vi "I64 to ZigZag.vi"(11 "sint64":i64) -> (3 "ZigZag I64":i64)   [LabVIEW 2020, in "LV-Proto.lvlib"]
uses:
  LV-Proto.lvlib
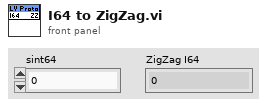
[diagram p1: front panel]
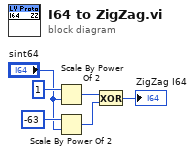
[diagram p0: block diagram]
diagram:
  n1 = Scale By Power Of 2(n=i16 1, x="sint64") -> (x*2^n=w3:i64)
  n2 = Scale By Power Of 2(n=i16 -63, x="sint64") -> (x*2^n=w2:i64)
  n3 = Exclusive Or(1:w2, 2:w3) -> (0:→"ZigZag I64":i64)
